vi "get_clock_params.vi"(8 "error in (no error)":errorcluster, 11 "Stimulator090724Scaffold in":refnum<class "Stimulator090724Scaffold.lvclass">) -> (0 "error out":errorcluster, 1 "repetitions":i32, 2 "duty cycle":dbl[unit], 3 "Stimulator090724Scaffold out":refnum<class "Stimulator090724Scaffold.lvclass">, 4 "frequency":dbl[unit], 5 "duration high":dbl[unit], 7 "offset":dbl[unit])   [LabVIEW 2010, in "Stimulator090724Scaffold.lvclass"]
uses:
  Stimulator090724Scaffold.lvclass
  Stimulator090724Scaffold.lvclass/Stimulator090724Scaffold.ctl
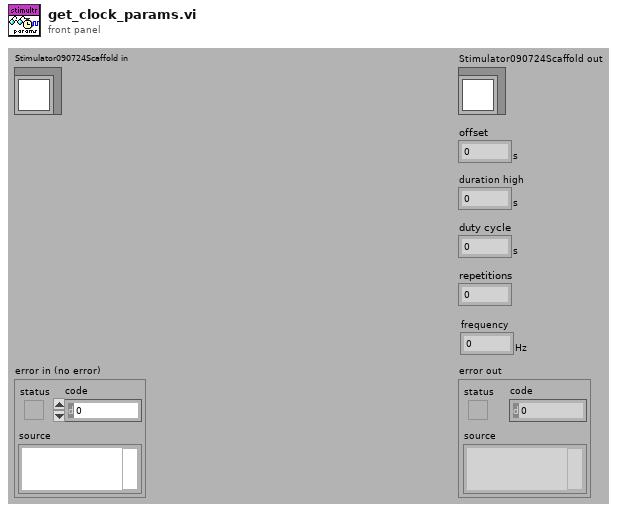
[diagram p1: front panel]
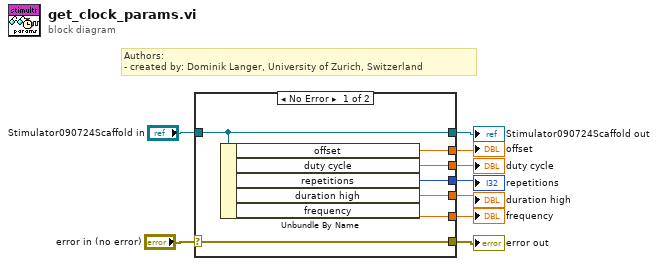
[diagram p0: block diagram]
diagram:
  # "Authors: \n- created by: Dominik Langer, University of Zurich, Switzerland"
  n1 = case shown="No Error" "error in (no error)" {
    selector: "error in (no error)" -> [w16 w18]
    tunnel: [w16 w18] -> w8
    tunnel: [w15 w17] -> w6
    tunnel: "Stimulator090724Scaffold in" -> [w15 w17]
    tunnel: [w14 _] -> w5
    tunnel: [w13 _] -> w4
    tunnel: [w12 _] -> w3
    tunnel: [w11 _] -> w2
    tunnel: [w10 _] -> w1
    frame No Error {
      n2 = Unbundle By Name(w15) -> ("offset"=w14:dbl[unit], "duty cycle"=w13:dbl[unit], "repetitions"=w12:i32, "duration high"=w11:dbl[unit], "frequency"=w10:dbl[unit])
    }
    frame Error {
    }
  }
  "error out" <- w8
  "Stimulator090724Scaffold out" <- w6
  "offset" <- w5
  "duty cycle" <- w4
  "repetitions" <- w3
  "duration high" <- w2
  "frequency" <- w1
